vi "Set Broadcast Message Transport.vi"(8 "error in (no error)":errorcluster, 10 "Broadcast Message Transport":refnum<class "Message Transport Queue.lvclass">, 11 "Websocket Topic Actor in":refnum<class "Websocket Topic Actor.lvclass">) -> (0 "error out":errorcluster, 3 "Websocket Topic Actor out":refnum<class "Websocket Topic Actor.lvclass">)   [LabVIEW 2016, in "Stream Mediator.lvlib" / "Websocket Topic Actor.lvclass"]
doc: "--\nCopyright © 2017 Composed SystemsI All rights reserved.\n\nAuthor: Jon McBee <jon.mcbee@composed.io>\n\nThis library is provided \"AS IS\" ,WITHOUT WARRANTIES OR\nCONDITIONS OF ANY KIND, either express or implied.\n\nComposed Systems -- composed.io\n\nStream 0.0.1.1\nJon McBee - Composed Systems\nCopyright (c) 2017, Composed Systems"
uses:
  <userlib>/Composed Systems/Stream/Mediator/Classes/Websocket Topic Actor/Websocket Topic Actor.lvclass
  <userlib>/Composed Systems/Stream/Mediator/Classes/Message Transport Queue/Message Transport Queue.lvclass
  <userlib>/Composed Systems/Stream/Mediator/Classes/Websocket Topic Actor/Websocket Topic Actor.lvclass/Websocket Topic Actor.ctl
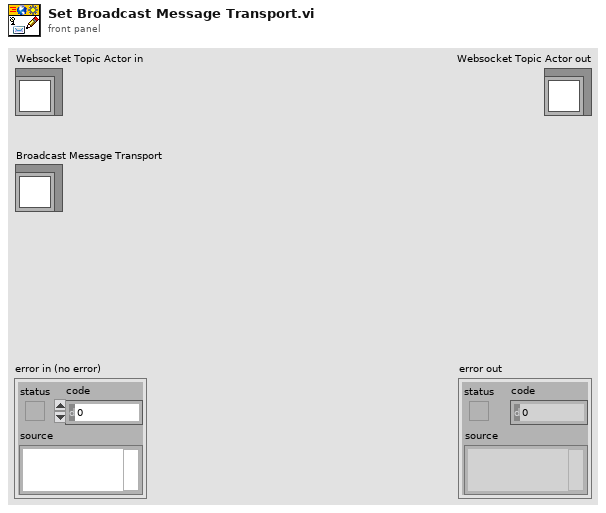
[diagram p1: front panel]
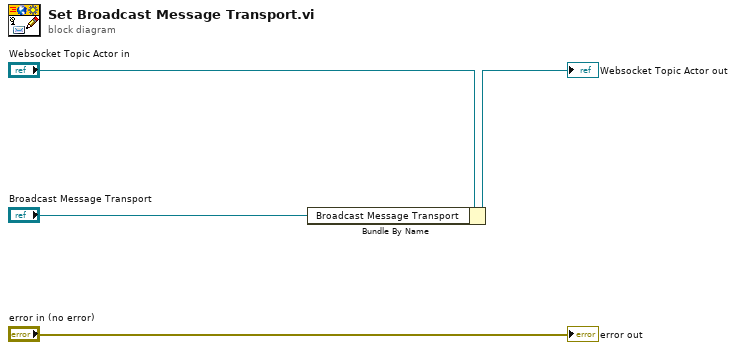
[diagram p0: block diagram]
diagram:
  n1 = Bundle By Name(cluster="Websocket Topic Actor in", "Broadcast Message Transport"="Broadcast Message Transport") -> (→"Websocket Topic Actor out":refnum<class "Websocket Topic Actor.lvclass">)
  "error out" <- "error in (no error)"
